vi "motorsGlobalVar.vi"() -> ()   [LabVIEW 2021]
panel:
  in  "GetPOS X":refnum<vi>
  in  "GetPOS Y":refnum<vi>
  in  "Don't Go Home":bool
  in  "Shutter toggle":bool
  in  "STOP application":bool
  in  "Motor Global Var":dbl[][](array[numeric]) format="%#_10g"
  # "These are absolute positions"
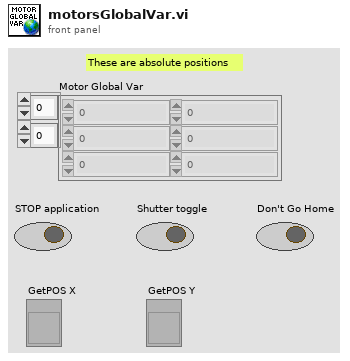
[diagram p1: front panel]
diagram:
